vi "Change Model File Path.vi"(7 "Model File Type":T1, 11 "Current Model":string) -> (2 "New Model path":path, 3 "New Model":string)   [LabVIEW 2015]
doc: "Change the path of the model being used based on the specified model type.\n____\nDelacor QMH Thermal Chamber Examples 4.0.0.21\nCopyright (c) 2018, Delacor"
uses:
  Model File Type--enum.ctl
panel:
  out "Current Model Path":path
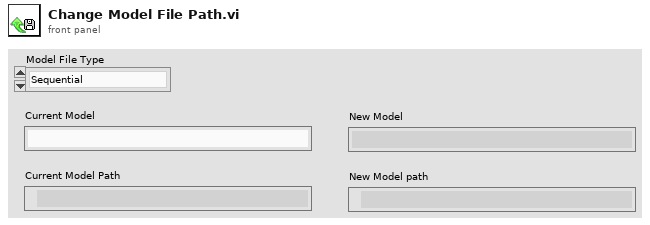
[diagram p1: front panel]
types:
  T1 = typedef "Model File Type--enum.ctl" = enum16{"Sequential", "Batch", "Parallel"}
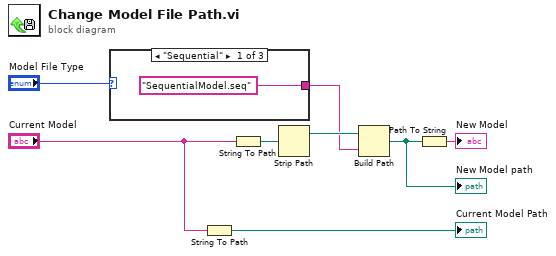
[diagram p0: block diagram]
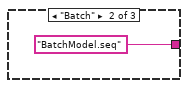
[diagram p2: hidden frame]
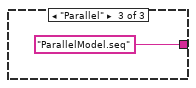
[diagram p3: hidden frame]
diagram:
  n1 = case shown="\"Sequential\"" "Model File Type" {
    tunnel: ["SequentialModel.seq" "BatchModel.seq" "ParallelModel.seq"] -> w1
    frame "Sequential" {
    }
    frame "Batch" {
    }
    frame "Parallel" {
    }
  }
  n2 = String To Path(string="Current Model") -> (path=→"Current Model Path":path)
  n3 = String To Path(string="Current Model") -> (path=w6:path)
  n4 = Strip Path(path=w6) -> (stripped path=w4:path)  [unwired: 1 out]
  n5 = Build Path(base path=w4, name or relative path=w1) -> (appended path=w2:path)
  "New Model path" <- w2
  n6 = Path To String(path=w2) -> (string=→"New Model":string)
